vi "main.vi"() -> ()   [LabVIEW 2010]
uses:
  <vilib>/Instr/_visa.llb/VISA Flush IO Buffer Mask.ctl
  <vilib>/Instr/_visa.llb/VISA Configure Serial Port (Instr).vi
panel:
  in  "Boolean":bool
  in  "Serial number:":u16=1 min=1
  in  "send 6":bool
  in  "send 4":bool
  in  "Screen bright:":u8 max=15 step=1
  out "Slide 2":dbl(slide) scale=0.0..1.0
  in  "Path to folder:":path
  in  "folder":bool
  in  "send 2":bool
  in  "Image index:":u8 max=127 step=1
  out "Slide":dbl(slide) scale=0.0..1.0
  out "error out":errorcluster
  in  "Path to bitmap file:":path
  out "TX = RX":bool
  out "TX = RX":bool[](array[boolean])
  out "bytes sent":u32
  in  "send":bool
  out "read":u8[](array[numeric])
  out "read":errorcluster
  out "return count":u32
  in  "Image index:":i32 max=127 step=1
  in  "Device COM port:":refnum<visa-resource-name>
  # "Max: 239"
  # "v1.1"
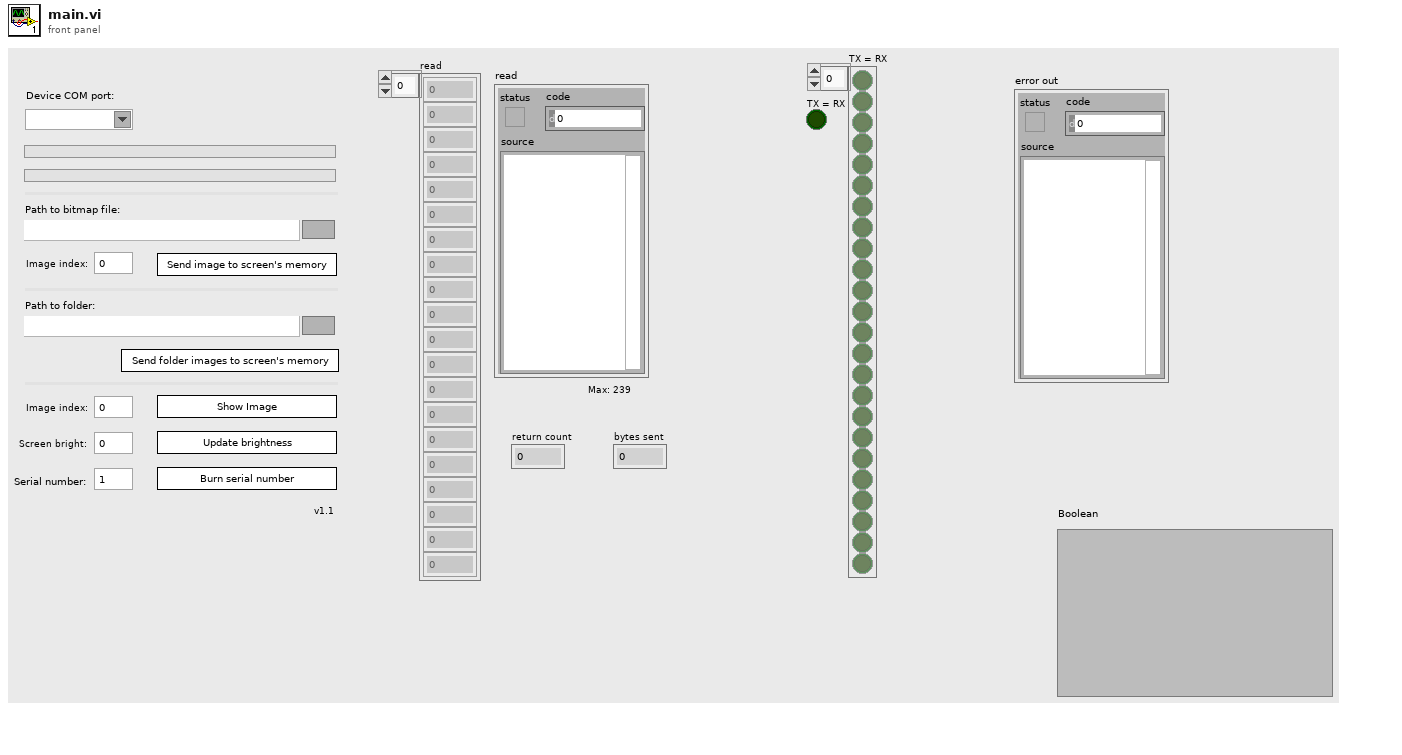
[diagram p1: front panel]
types:
  T1 = typedef "VISA Flush IO Buffer Mask.ctl" = u16
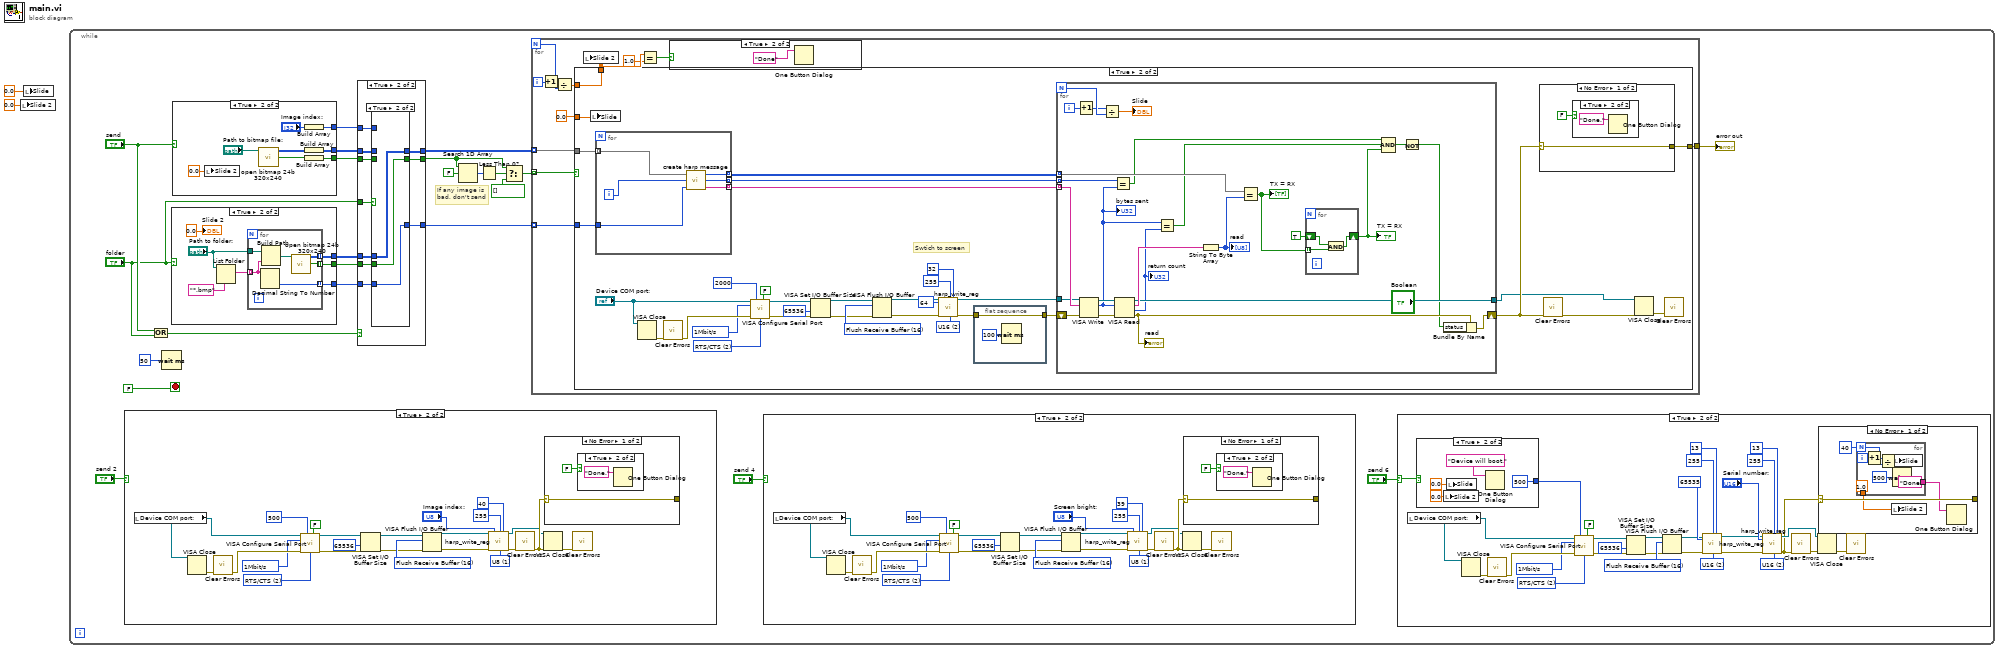
[diagram p0: block diagram]
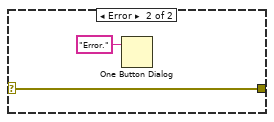
[diagram p4: hidden frame]
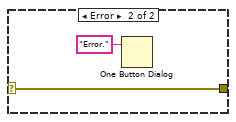
[diagram p7: hidden frame]
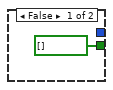
[diagram p8: hidden frame]
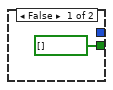
[diagram p10: hidden frame]
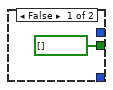
[diagram p11: hidden frame]
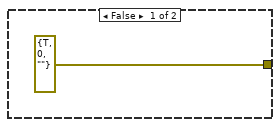
[diagram p13: hidden frame]
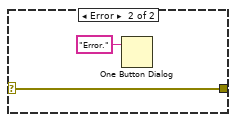
[diagram p15: hidden frame]
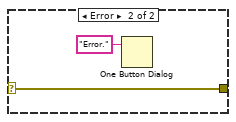
[diagram p18: hidden frame]
diagram:
  n1 = local write "Slide 2"(0.0 ("Slide 2")) -> ()
  n2 = local write "Slide"(0.0 ("Slide 2")) -> ()
  n3 = while {
    stop <- FALSE ("stop") stop-if-true
    # "If any image is\nbad, don't send"
    n4 = case shown="True" "send 2" {
      frame False {
      }
      frame True {
        w238 = u8 1 items=["U8"=1, "U16"=2, "U32"=4, "U64"=8, "I8"=129, "I16"=130, "I32"=132, "I64"=136, "FLOAT"=68, "BOOL"=17] ("type")
        w243 = T1 16 items=["Flush Receive Buffer"=16, "Write Transmit Buffer to Device"=32, "Flush Receive Buffer (No I/O)"=64, "Flush Transmit Buffer"=128] ("Mask")
        w247 = u32 1000000 items=["250Kbit/s"=250000, "500kbit/s"=500000, "1Mbit/s"=1000000, "2Mbit/s"=2000000, "4Mbit/s"=4000000] ("baud rate")
        w248 = u16 2 items=["None", "XON/XOFF", "RTS/CTS", "XON/XOFF & RTS/CTS", "DTR/DSR", "XON/XOFF & DTR/DSR"] ("flow control (0:none)")
        n5 = local read "Device COM port:"() -> (w230:refnum<visa-resource-name>)
        n6 = VISA Close(VISA resource name=w230) -> (error out=w249:errorcluster)  [unwired: 1 in]
        n7 = call <vilib>:"Clear Errors.vi"("error in (no error)"=w249) -> ("error out"=w251:errorcluster)  [unwired: 6 in]
        n8 = call-poly "VISA Configure Serial Port"("VISA resource name"=w230, "timeout (10sec)"=u32 500, "Enable Termination\nChar (T)"=FALSE ("Enable Termination\nChar (T)"), "baud rate (9600)"=w247, "error in (no error)"=w251, "flow control (0:none)"=w248) -> ("VISA resource name out"=w245:refnum<visa-resource-name>, "error out"=w246:errorcluster)  [unwired: 8 in]
        n9 = VISA Set I/O Buffer Size(VISA resource name=w245, size (4096)=u32 65536, error in (no error)=w246) -> (VISA resource name out=w241:refnum<visa-resource-name>, error out=w242:errorcluster)  [unwired: 1 in]
        n10 = VISA Flush I/O Buffer(VISA resource name=w241, mask (16)=w243, error in (no error)=w242) -> (VISA resource name out=w239:refnum<visa-resource-name>, error out=w240:errorcluster)
        n11 = call "harp_write_reg.vi"(0:"port"=w239, "error in (no error)"=w240, "8 bits"="Image index:", 10:"port"=u8 255 ("port"), "type"=w238, "reg. address"=u8 40) -> ("port out"=w231:refnum<visa-resource-name>, "error out"=w234:errorcluster)  [unwired: 11 in, 1 out]
        n12 = call <vilib>:"Clear Errors.vi"("error in (no error)"=w234) -> ("error out"=w233:errorcluster)  [unwired: 6 in]
        n13 = VISA Close(VISA resource name=w231, error in (no error)=w233) -> (error out=w235:errorcluster)
        n14 = case shown="No Error" w233 {
          selector: w233 -> [w254 w256]
          tunnel: [w254 w256] -> _
          frame No Error {
            n15 = case shown="True" FALSE {
              frame False {
              }
              frame True {
                n16 = One Button Dialog(message="Done.") -> ()  [unwired: 1 in, 1 out]
              }
            }
          }
          frame Error {
            n17 = One Button Dialog(message="Error.") -> ()  [unwired: 1 in, 1 out]
          }
        }
        n18 = call <vilib>:"Clear Errors.vi"("error in (no error)"=w235) -> ()  [unwired: 6 in, 1 out]
      }
    }
    n19 = Or(x="send", y="folder") -> (x .or. y?=w11:bool)
    n20 = Wait (ms)(milliseconds to wait=u32 50) -> ()  [unwired: 1 out]
    n21 = case shown="True" "folder" {
      tunnel: [_ w131] -> w19
      tunnel: [bool[] [] w130] -> w18
      tunnel: [_ w129] -> w17
      frame False {
      }
      frame True {
        n22 = List Folder(path="Path to folder:", pattern="*.bmp") -> (filenames=w132:string[])  [unwired: 2 in, 3 out]
        n23 = for {
          tunnel: w132 -> [w139] mode=indexing
          tunnel: [w140] -> w129 mode=indexing
          tunnel: "Path to folder:" -> [w138]
          tunnel: [w136] -> w131 mode=indexing
          tunnel: [w135] -> w130 mode=indexing
          n24 = Decimal String To Number(string=w139) -> (number=w140:i32)  [unwired: 2 in, 1 out]
          n25 = Build Path(base path=w138, name or relative path=w139) -> (appended path=w137:path)
          n26 = call "open bitmap 24b 320x240.vi"("path to BMP file"=w137) -> ("raw data"=w136:u16[][], "image ok"=w135:bool)  [unwired: 13 in]
        }
        "Slide 2" <- 0.0 ("Slide 2")
      }
    }
    n27 = case shown="True" "send" {
      tunnel: [_ w124] -> w16
      tunnel: [bool[] [] w122] -> w15
      tunnel: [_ w120] -> w14
      frame False {
      }
      frame True {
        n28 = local write "Slide 2"(0.0 ("Slide 2")) -> ()
        n29 = call "open bitmap 24b 320x240.vi"("path to BMP file"="Path to bitmap file:") -> ("raw data"=w126:u16[][], "image ok"=w123:bool)  [unwired: 13 in]
        n30 = Build Array(w126) -> (w124:u16[][][])
        n31 = Build Array(w123) -> (w122:bool[])
        n32 = Build Array("Image index:") -> (w120:i32[])
      }
    }
    n33 = case shown="True" w11 {
      tunnel: [_ w111] -> w23
      tunnel: [bool[] [] w110] -> w7
      tunnel: [_ w109] -> w20
      tunnel: "folder" -> [_ w108]
      tunnel: w19 -> [_ w107]
      tunnel: w18 -> [_ w106]
      tunnel: w17 -> [_ w105]
      tunnel: w16 -> [_ w104]
      tunnel: w15 -> [_ w103]
      tunnel: w14 -> [_ w102]
      frame False {
      }
      frame True {
        n34 = case shown="True" w108 {
          tunnel: w107 -> [_ w117]
          tunnel: w106 -> [_ w116]
          tunnel: w105 -> [_ w115]
          tunnel: w104 -> [w114 _]
          tunnel: w103 -> [w113 _]
          tunnel: [w114 w117] -> w111
          tunnel: [w113 w116] -> w110
          tunnel: [w112 w115] -> w109
          tunnel: w102 -> [w112 _]
          frame False {
          }
          frame True {
          }
        }
      }
    }
    n35 = Search 1D Array(1D array=w7, element=FALSE) -> (index of element=w9:i32)  [unwired: 1 in]
    n36 = Less Than 0?(x=w9) -> (x < 0?=w8:bool)
    n37 = Select(t=w7, s=w8, f=bool[] []) -> (s? t:f=w5:bool[])
    n38 = for {
      N -> [w145]
      tunnel: w23 -> [w152] mode=indexing
      tunnel: w5 -> [w151] mode=indexing
      tunnel: [w150] -> w22
      tunnel: w20 -> [w149] mode=indexing
      i -> [w146]
      n39 = Increment(x=w146) -> (x+1=w147:i32)
      n40 = Divide(x=w147, y=w145) -> (x/y=w144:dbl)
      n41 = case shown="True" w151 {
        tunnel: w152 -> [_ w175]
        tunnel: [errorcluster {"status"=TRUE, "code"=0, "source"=""} ("error IO") w161] -> w150
        tunnel: w149 -> [_ w157]
        tunnel: 0.0 ("Slide") -> [_ w156]
        tunnel: [_ w155] -> w143
        tunnel: w144 -> [_ w155]
        frame False {
        }
        frame True {
          w169 = u8 2 items=["U8"=1, "U16"=2, "U32"=4, "U64"=8, "I8"=129, "I16"=130, "I32"=132, "I64"=136, "FLOAT"=68, "BOOL"=17] ("type")
          w179 = T1 16 items=["Flush Receive Buffer"=16, "Write Transmit Buffer to Device"=32, "Flush Receive Buffer (No I/O)"=64, "Flush Transmit Buffer"=128] ("Mask")
          w183 = u32 1000000 items=["250Kbit/s"=250000, "500kbit/s"=500000, "1Mbit/s"=1000000, "2Mbit/s"=2000000, "4Mbit/s"=4000000] ("baud rate")
          w184 = u16 2 items=["None", "XON/XOFF", "RTS/CTS", "XON/XOFF & RTS/CTS", "DTR/DSR", "XON/XOFF & DTR/DSR"] ("flow control (0:none)")
          # "Swtich to screen"
          n42 = local write "Slide"(w156) -> ()
          n43 = for {
            tunnel: w175 -> [w229] mode=indexing
            tunnel: [w228] -> w174 mode=indexing
            tunnel: [w227] -> w173 mode=indexing
            tunnel: [w226] -> w172 mode=indexing
            tunnel: w157 -> [w224]
            i -> [w225]
            n44 = call "create harp message.vi"("image index"=w224, "column index (0-319)"=w225, "column data"=w229) -> (0:"U8 Array to send"=w228:string, "harp message size"=w227:i32, 2:"U8 Array to send"=w226:u8[])
          }
          n45 = VISA Close(VISA resource name="Device COM port:") -> (error out=w185:errorcluster)  [unwired: 1 in]
          n46 = call <vilib>:"Clear Errors.vi"("error in (no error)"=w185) -> ("error out"=w187:errorcluster)  [unwired: 6 in]
          n47 = call-poly "VISA Configure Serial Port"("VISA resource name"="Device COM port:", "timeout (10sec)"=u32 2000, "Enable Termination\nChar (T)"=FALSE ("Enable Termination\nChar (T)"), "baud rate (9600)"=w183, "error in (no error)"=w187, "flow control (0:none)"=w184) -> ("VISA resource name out"=w181:refnum<visa-resource-name>, "error out"=w182:errorcluster)  [unwired: 8 in]
          n48 = VISA Set I/O Buffer Size(VISA resource name=w181, size (4096)=u32 65536, error in (no error)=w182) -> (VISA resource name out=w177:refnum<visa-resource-name>, error out=w178:errorcluster)  [unwired: 1 in]
          n49 = VISA Flush I/O Buffer(VISA resource name=w177, mask (16)=w179, error in (no error)=w178) -> (VISA resource name out=w170:refnum<visa-resource-name>, error out=w171:errorcluster)
          n50 = call "harp_write_reg.vi"(0:"port"=w170, "16 bits"=u16 64, "error in (no error)"=w171, 10:"port"=u8 255 ("port"), "type"=w169, "reg. address"=u8 32) -> ("port out"=w165:refnum<visa-resource-name>, "error out"=w164:errorcluster)  [unwired: 11 in, 1 out]
          n51 = flat-sequence {
            tunnel: w164 -> [w195]
            tunnel: [w195] -> w163
            frame #0 {
              n52 = Wait (ms)(milliseconds to wait=u32 100) -> ()  [unwired: 1 out]
            }
          }
          n53 = for {
            N -> [w198]
            tunnel: w174 -> [w213] mode=indexing
            tunnel: [w212] -> w159
            shift-right: [w203] -> w162
            shift-left: w163 -> [w214]
            tunnel: w173 -> [w211] mode=indexing
            tunnel: w172 -> [w208] mode=indexing
            tunnel: w165 -> [w200]
            i -> [w199]
            n54 = Increment(x=w199) -> (x+1=w197:i32)
            n55 = VISA Write(VISA resource name=w200, write buffer=w213, error in (no error)=w214) -> (VISA resource name out=w219:refnum<visa-resource-name>, return count=w209:u32, error out=w220:errorcluster)
            "bytes sent" <- w209
            n56 = Divide(x=w197, y=w198) -> (x/y=→"Slide":dbl)
            n57 = Equal?(x=w211, y=w209) -> (x = y?=w205:bool)
            n58 = VISA Read(VISA resource name=w219, byte count=w209, error in (no error)=w220) -> (VISA resource name out=w212:refnum<visa-resource-name>, read buffer=w218:string, return count=w210:u32, error out=w204:errorcluster)
            "return count" <- w210
            "read" <- w204
            n59 = Equal?(x=w209, y=w210) -> (x = y?=w206:bool)
            n60 = String To Byte Array(string=w218) -> (unsigned byte array=w217:u8[])
            "read" <- w217
            n61 = Equal?(x=w208, y=w217) -> (x = y?=w216:bool[])
            "TX = RX" <- w216
            n62 = for {
              shift-right: [w222] -> w207
              shift-left: TRUE -> [w221]
              tunnel: w216 -> [w223] mode=indexing
              n63 = And(x=w221, y=w223) -> (x .and. y?=w222:bool)
            }
            "TX = RX" <- w207
            n64 = Compound Arithmetic op=AND(w205, w206, w207) -> (w202:bool)
            n65 = Not(x=w202) -> (.not. x?=w201:bool)
            n66 = Bundle By Name(cluster=w204, "status"=w201) -> (w203:errorcluster)
          }
          n67 = case shown="No Error" w162 {
            selector: w162 -> [w190 w192]
            tunnel: [w190 w192] -> w161
            frame No Error {
              n68 = case shown="True" FALSE {
                frame False {
                }
                frame True {
                  n69 = One Button Dialog(message="Done.") -> ()  [unwired: 1 in, 1 out]
                }
              }
            }
            frame Error {
              n70 = One Button Dialog(message="Error.") -> ()  [unwired: 1 in, 1 out]
            }
          }
          n71 = call <vilib>:"Clear Errors.vi"("error in (no error)"=w162) -> ("error out"=w158:errorcluster)  [unwired: 6 in]
          n72 = VISA Close(VISA resource name=w159, error in (no error)=w158) -> (error out=w160:errorcluster)
          n73 = call <vilib>:"Clear Errors.vi"("error in (no error)"=w160) -> ()  [unwired: 6 in, 1 out]
        }
      }
      n74 = local write "Slide 2"(w143) -> ()
      n75 = Equal?(x=w143, y=1.0) -> (x = y?=w141:bool)
      n76 = case shown="True" w141 {
        frame False {
        }
        frame True {
          n77 = One Button Dialog(message="Done") -> ()  [unwired: 1 in, 1 out]
        }
      }
    }
    "error out" <- w22
    n78 = case shown="True" "send 4" {
      frame False {
      }
      frame True {
        w81 = u8 1 items=["U8"=1, "U16"=2, "U32"=4, "U64"=8, "I8"=129, "I16"=130, "I32"=132, "I64"=136, "FLOAT"=68, "BOOL"=17] ("type")
        w86 = T1 16 items=["Flush Receive Buffer"=16, "Write Transmit Buffer to Device"=32, "Flush Receive Buffer (No I/O)"=64, "Flush Transmit Buffer"=128] ("Mask")
        w90 = u32 1000000 items=["250Kbit/s"=250000, "500kbit/s"=500000, "1Mbit/s"=1000000, "2Mbit/s"=2000000, "4Mbit/s"=4000000] ("baud rate")
        w91 = u16 2 items=["None", "XON/XOFF", "RTS/CTS", "XON/XOFF & RTS/CTS", "DTR/DSR", "XON/XOFF & DTR/DSR"] ("flow control (0:none)")
        n79 = local read "Device COM port:"() -> (w74:refnum<visa-resource-name>)
        n80 = VISA Close(VISA resource name=w74) -> (error out=w92:errorcluster)  [unwired: 1 in]
        n81 = call <vilib>:"Clear Errors.vi"("error in (no error)"=w92) -> ("error out"=w94:errorcluster)  [unwired: 6 in]
        n82 = call-poly "VISA Configure Serial Port"("VISA resource name"=w74, "timeout (10sec)"=u32 500, "Enable Termination\nChar (T)"=FALSE ("Enable Termination\nChar (T)"), "baud rate (9600)"=w90, "error in (no error)"=w94, "flow control (0:none)"=w91) -> ("VISA resource name out"=w88:refnum<visa-resource-name>, "error out"=w89:errorcluster)  [unwired: 8 in]
        n83 = VISA Set I/O Buffer Size(VISA resource name=w88, size (4096)=u32 65536, error in (no error)=w89) -> (VISA resource name out=w84:refnum<visa-resource-name>, error out=w85:errorcluster)  [unwired: 1 in]
        n84 = VISA Flush I/O Buffer(VISA resource name=w84, mask (16)=w86, error in (no error)=w85) -> (VISA resource name out=w82:refnum<visa-resource-name>, error out=w83:errorcluster)
        n85 = call "harp_write_reg.vi"(0:"port"=w82, "error in (no error)"=w83, "8 bits"="Screen bright:", 10:"port"=u8 255 ("port"), "type"=w81, "reg. address"=u8 39) -> ("port out"=w75:refnum<visa-resource-name>, "error out"=w77:errorcluster)  [unwired: 11 in, 1 out]
        n86 = call <vilib>:"Clear Errors.vi"("error in (no error)"=w77) -> ("error out"=w76:errorcluster)  [unwired: 6 in]
        n87 = VISA Close(VISA resource name=w75, error in (no error)=w76) -> (error out=w78:errorcluster)
        n88 = case shown="No Error" w76 {
          selector: w76 -> [w97 w99]
          tunnel: [w97 w99] -> _
          frame No Error {
            n89 = case shown="True" FALSE {
              frame False {
              }
              frame True {
                n90 = One Button Dialog(message="Done.") -> ()  [unwired: 1 in, 1 out]
              }
            }
          }
          frame Error {
            n91 = One Button Dialog(message="Error.") -> ()  [unwired: 1 in, 1 out]
          }
        }
        n92 = call <vilib>:"Clear Errors.vi"("error in (no error)"=w78) -> ()  [unwired: 6 in, 1 out]
      }
    }
    n93 = case shown="True" "send 6" {
      selector: "send 6" -> [_ w36]
      frame False {
      }
      frame True {
        w31 = u8 2 items=["U8"=1, "U16"=2, "U32"=4, "U64"=8, "I8"=129, "I16"=130, "I32"=132, "I64"=136, "FLOAT"=68, "BOOL"=17] ("type")
        w44 = u8 2 items=["U8"=1, "U16"=2, "U32"=4, "U64"=8, "I8"=129, "I16"=130, "I32"=132, "I64"=136, "FLOAT"=68, "BOOL"=17] ("type")
        w47 = T1 16 items=["Flush Receive Buffer"=16, "Write Transmit Buffer to Device"=32, "Flush Receive Buffer (No I/O)"=64, "Flush Transmit Buffer"=128] ("Mask")
        w51 = u32 1000000 items=["250Kbit/s"=250000, "500kbit/s"=500000, "1Mbit/s"=1000000, "2Mbit/s"=2000000, "4Mbit/s"=4000000] ("baud rate")
        w52 = u16 2 items=["None", "XON/XOFF", "RTS/CTS", "XON/XOFF & RTS/CTS", "DTR/DSR", "XON/XOFF & DTR/DSR"] ("flow control (0:none)")
        n94 = local read "Device COM port:"() -> (w38:refnum<visa-resource-name>)
        n95 = case shown="True" w36 {
          tunnel: [_ u32 500 ("timeout (10sec)")] -> w35
          frame False {
          }
          frame True {
            n96 = local write "Slide 2"(0.0 ("Slide")) -> ()
            n97 = local write "Slide"(0.0 ("Slide")) -> ()
            n98 = One Button Dialog(message="Device will boot.") -> ()  [unwired: 1 in, 1 out]
          }
        }
        n99 = VISA Close(VISA resource name=w38) -> (error out=w53:errorcluster)  [unwired: 1 in]
        n100 = call <vilib>:"Clear Errors.vi"("error in (no error)"=w53) -> ("error out"=w54:errorcluster)  [unwired: 6 in]
        n101 = call-poly "VISA Configure Serial Port"("VISA resource name"=w38, "timeout (10sec)"=w35, "Enable Termination\nChar (T)"=FALSE ("Enable Termination\nChar (T)"), "baud rate (9600)"=w51, "error in (no error)"=w54, "flow control (0:none)"=w52) -> ("VISA resource name out"=w49:refnum<visa-resource-name>, "error out"=w50:errorcluster)  [unwired: 8 in]
        n102 = VISA Set I/O Buffer Size(VISA resource name=w49, size (4096)=u32 65536, error in (no error)=w50) -> (VISA resource name out=w45:refnum<visa-resource-name>, error out=w46:errorcluster)  [unwired: 1 in]
        n103 = VISA Flush I/O Buffer(VISA resource name=w45, mask (16)=w47, error in (no error)=w46) -> (VISA resource name out=w30:refnum<visa-resource-name>, error out=w27:errorcluster)
        n104 = call "harp_write_reg.vi"(0:"port"=w30, "16 bits"=u16 65535 ("Serial number: 2"), "error in (no error)"=w27, 10:"port"=u8 255 ("port"), "type"=w31, "reg. address"=u8 13) -> ("port out"=w29:refnum<visa-resource-name>, "error out"=w26:errorcluster)  [unwired: 11 in, 1 out]
        n105 = call "harp_write_reg.vi"(0:"port"=w29, "16 bits"="Serial number:", "error in (no error)"=w26, 10:"port"=u8 255 ("port"), "type"=w44, "reg. address"=u8 13) -> ("port out"=w39:refnum<visa-resource-name>, "error out"=w28:errorcluster)  [unwired: 11 in, 1 out]
        n106 = call <vilib>:"Clear Errors.vi"("error in (no error)"=w28) -> ("error out"=w40:errorcluster)  [unwired: 6 in]
        n107 = VISA Close(VISA resource name=w39, error in (no error)=w40) -> (error out=w41:errorcluster)
        n108 = case shown="No Error" w28 {
          selector: w28 -> [w63 w71]
          tunnel: [w63 w71] -> _
          frame No Error {
            n109 = for {
              N: 40 -> [w69]
              tunnel: [1.0 ("Slide 2")] -> w61
              tunnel: ["Done" ("message")] -> w60
              i -> [w70]
              n110 = Increment(x=w70) -> (x+1=w68:i32)
              n111 = Divide(x=w68, y=w69) -> (x/y=w67:dbl)
              n112 = local write "Slide"(w67) -> ()
              n113 = Wait (ms)(milliseconds to wait=u32 500) -> ()  [unwired: 1 out]
            }
            n114 = local write "Slide 2"(w61) -> ()
            n115 = One Button Dialog(message=w60) -> ()  [unwired: 1 in, 1 out]
          }
          frame Error {
            n116 = One Button Dialog(message="Error.") -> ()  [unwired: 1 in, 1 out]
          }
        }
        n117 = call <vilib>:"Clear Errors.vi"("error in (no error)"=w41) -> ()  [unwired: 6 in, 1 out]
      }
    }
  }
